vi "CRYStep Setup Default Window.vi"() -> ()   [LabVIEW 2013]
uses:
  CRYWindow/SubVI/CRYMain Sub Window Global.vi
panel:
  in  "Curve Change":enum16{"Curves", "Values", "Results", "WFM"}[](array[ring])
  in  "stop":bool
  out "DefaultEmptyStep":string="\nGVSoundLab!\n\nThis Window is Step Setup Editor Window.\nPlease, Select any step in Project Window."
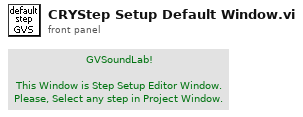
[diagram p1: front panel]
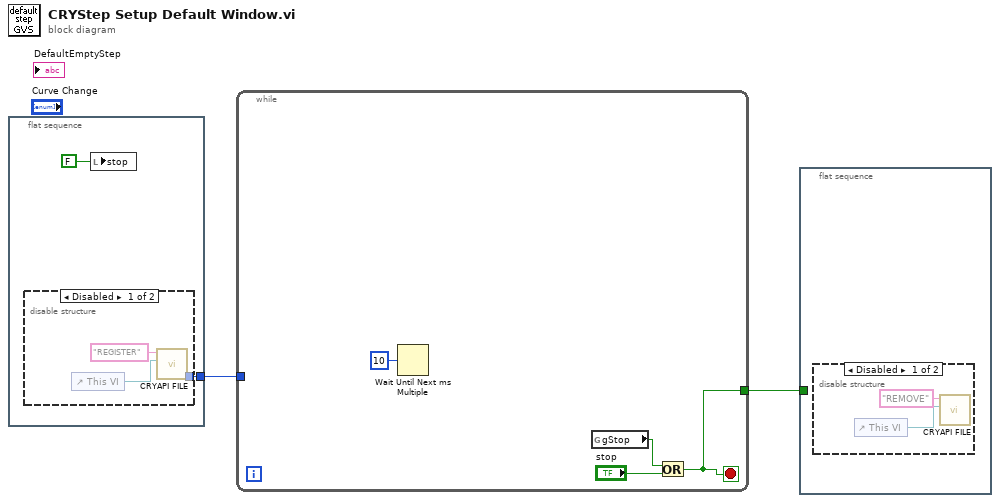
[diagram p0: block diagram]
diagram:
  n1 = flat-sequence {
    tunnel: [w4] -> w2
    frame #0 {
      n2 = disable-structure shown="Disabled" {
        disable-tunnel: [w5 _] -> w4
        frame Disabled {
          n3 = control-ref of="This VI"() -> (w6:refnum<vi>)
          n4 = call "CRYAPI FILE.vi"("pVIRef"=w6, "sAction"="REGISTER") -> ("nData_Out"=w5:i32)  [unwired: 8 in, 1 out]
        }
        frame Enabled {
        }
      }
      n5 = local write "stop"(FALSE ("stop")) -> ()
    }
  }
  n6 = while {
    tunnel: w2 -> [_]
    tunnel: [w9] -> w1
    stop <- w9 stop-if-true
    n7 = Wait Until Next ms Multiple(millisecond multiple=u32 10) -> ()  [unwired: 1 out]
    n8 = global read "CRYMain Sub Window Global.vi" "gStop"() -> (w11:bool)
    n9 = Or(x=w11, y="stop") -> (x .or. y?=w9:bool)
  }
  n10 = flat-sequence {
    tunnel: w1 -> [_]
    frame #0 {
      n11 = disable-structure shown="Disabled" {
        frame Disabled {
          n12 = control-ref of="This VI"() -> (w12:refnum<vi>)
          n13 = call "CRYAPI FILE.vi"("pVIRef"=w12, "sAction"="REMOVE") -> ()  [unwired: 8 in, 2 out]
        }
        frame Enabled {
        }
      }
    }
  }
